vi "DP-Init Raw Data File.vi"(0 "state":T2, 7 "level series in":T1, 11 "error in (no error)":errorcluster) -> (8 "level series out":T1, 15 "error out":errorcluster)   [LabVIEW 2020]
uses:
  Typedefs/DP-Runtime State.ctl
  Typedefs/DP-Level Series Info.ctl
  Typedefs/DP-Raw Data Header.ctl
  42e42a8b-3526-40fb-97e3-6616fd7f9e9f.vi
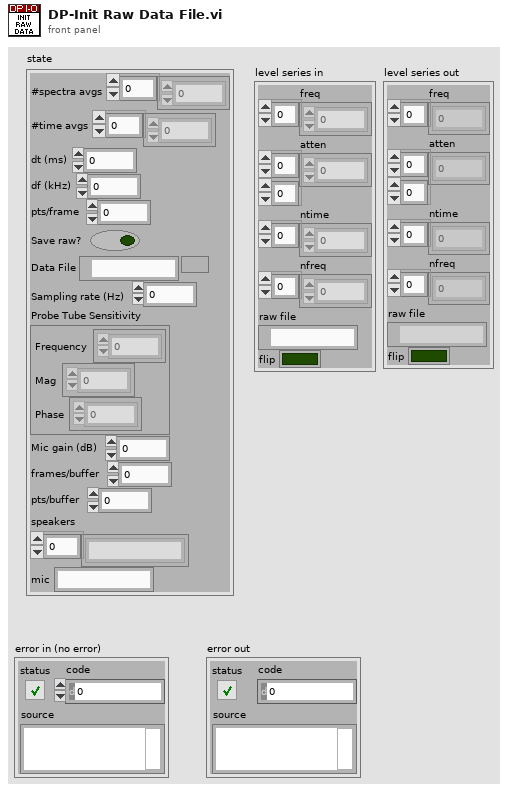
[diagram p1: front panel]
types:
  T1 = typedef "DP-Level Series Info.ctl" = cluster{"freq":dbl[], "atten":dbl[][], "ntime":i32[], "nfreq":i32[], "raw file":path, "flip":bool}
  T2 = typedef "DP-Runtime State.ctl" = cluster{"#spectra avgs":i32[], "#time avgs":i32[], "dt (ms)":dbl, "df (kHz)":dbl, "pts/frame":i32, "Save raw?":bool, "Data File":path, "Sampling rate (Hz)":dbl, "Probe Tube Sensitivity":cluster{"Frequency":dbl[], "Mag":dbl[], "Phase":dbl[]}, "Mic gain (dB)":dbl, "frames/buffer":i32, "pts/buffer":i32, "speakers":string[], "mic":string}
  T3 = typedef "DP-Raw Data Header.ctl" = cluster{"Probe Tube Sensitivity":cluster{"Frequency":dbl[], "Mag":dbl[], "Phase":dbl[]}, "Mic gain (dB)":dbl, "Sampling rate (Hz)":dbl, "pts/frame":i32, "frames/buffer":i32, "pts/buffer":i32}
  T4 = enum16{"open", "replace", "create", "open or create", "replace or create", "replace or create with confirmation"}
  T5 = cluster{"Frequency":dbl[], "Mag":dbl[], "Phase":dbl[]}
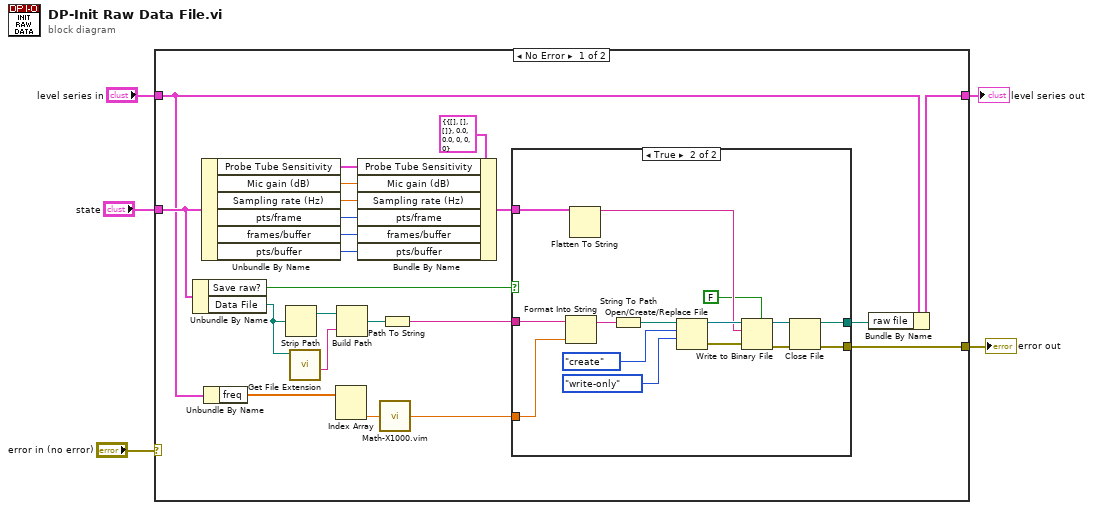
[diagram p0: block diagram]
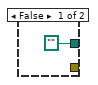
[diagram p2: hidden frame]
diagram:
  n1 = case shown="No Error" "error in (no error)" {
    selector: "error in (no error)" -> [_ w45]
    tunnel: "state" -> [w16 _]
    tunnel: [w26 w45] -> w4
    tunnel: "level series in" -> [w8 w44]
    tunnel: [w6 w44] -> w1
    frame No Error {
      n2 = Unbundle By Name(w16) -> ("Save raw?"=w18:bool, "Data File"=w22:path)
      n3 = Unbundle By Name(w16) -> ("Probe Tube Sensitivity"=w15:T5, "Mic gain (dB)"=w14:dbl, "Sampling rate (Hz)"=w13:dbl, "pts/frame"=w12:i32, "frames/buffer"=w11:i32, "pts/buffer"=w10:i32)
      n4 = Unbundle By Name(w8) -> ("freq"=w25:dbl[])
      n5 = Strip Path(path=w22) -> (stripped path=w21:path)  [unwired: 1 out]
      n6 = call <vilib>:"Get File Extension.vi"("file"=w22) -> ("filename without extension"=w20:string)  [unwired: 6 in, 4 out]
      n7 = Index Array(array=w25) -> (element #2=w24:dbl)  [unwired: 2 in, 1 out]
      n8 = Build Path(base path=w21, name or relative path=w20) -> (appended path=w19:path)
      n9 = Bundle By Name(cluster=T3 {"Probe Tube Sensitivity"={"Frequency"=[], "Mag"=[], "Phase"=[]}, "Mic gain (dB)"=0.0, "Sampling rate (Hz)"=0.0, "pts/frame"=0, "frames/buffer"=0, "pts/buffer"=0} ("header"), "Probe Tube Sensitivity"=w15, "Mic gain (dB)"=w14, "Sampling rate (Hz)"=w13, "pts/frame"=w12, "frames/buffer"=w11, "pts/buffer"=w10) -> (w9:T3)
      n10 = call "Math-X1000.vim"("X"=w24) -> ("1000X"=w23:dbl)
      n11 = Path To String(path=w19) -> (string=w27:string)
      n12 = case shown="True" w18 {
        tunnel: w27 -> [_ w41]
        tunnel: [path "" w33] -> w7
        tunnel: [_ w32] -> w26
        tunnel: w23 -> [_ w36]
        tunnel: w9 -> [_ w31]
        frame False {
        }
        frame True {
          n13 = Format Into String(initial string=w41, w36) -> (resulting string=w43:string)  [unwired: 2 in, 1 out]
          n14 = Flatten To String(anything=w31) -> (data string=w30:string)  [unwired: 3 in, 2 out]
          n15 = String To Path(string=w43) -> (path=w42:path)
          n16 = Open/Create/Replace File(file path (use dialog)=w42, operation (0:open)=T4."create", access (0:read/write)=enum16{"read/write", "read-only", "write-only"}."write-only") -> (refnum out=w39:refnum<file>, error out=w40:errorcluster)  [unwired: 3 in, 1 out]
          n17 = Write to Binary File(file (use dialog)=w39, data=w30, error in=w40, 5:FALSE ("prepend array or string size? (T)")) -> (refnum out=w34:refnum<file>, error out=w35:errorcluster)  [unwired: 2 in, 1 out]
          n18 = Close File(refnum=w34, error in=w35) -> (path=w33:path, error out=w32:errorcluster)
        }
      }
      n19 = Bundle By Name(cluster=w8, "raw file"=w7) -> (w6:T1)
    }
    frame Error {
    }
  }
  "error out" <- w4
  "level series out" <- w1
